vi "Pinholes.vi"(4 "Current Threshold [nA]":dbl, 5 "settling\ndelay":i32) -> (1 "excluded channels":i32[](array[numeric]), 2 "Current [nA]":dbl[](array[numeric]), 3 "Flag":i32[](array[numeric]))   [LabVIEW 2019]
uses:
  general_VIs/globals/QC_MeasurementSetup.vi
  InstrControl/Switching/Switching.lvclass
  InstrControl/SupplyControl/SupplyControl.lvclass
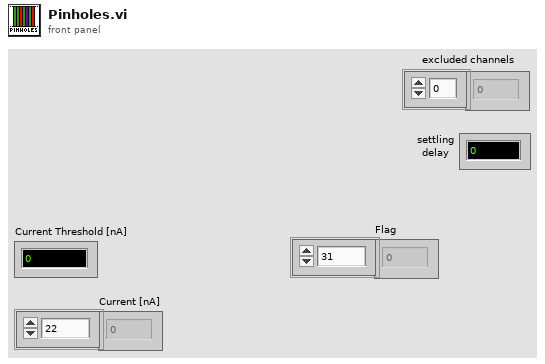
[diagram p1: front panel]
types:
  T1 = cluster{"Bias Supply":refnum<class "SupplyControl.lvclass">, "SMU":refnum<class "SupplyControl.lvclass">, "LCR":refnum<class "LCRControl.lvclass">, "Probe Card Channels":i32, "Bias Voltage [V]":dbl, "First strip":i32, "Last strip":i32, "Base Voltage [V]":dbl, "Base Ramp Step [V]":dbl, "Base Ramp Interval [ms]":u32, "High Voltage [V]":dbl, "High Ramp Step [V]":dbl, "High Ramp Interval [ms]":u32, "AC frequency [Hz]":i32, "AC amplitude [V]":dbl, "RC Configuration":u16, "Single Needle":bool, "Temperature Readout":enum16{"Read Arduino", "Enter manually"}, "Arduino":refnum<class "ArduinoControl.lvclass">, "Fraction of good strips [%]":dbl, "ProbeStation":refnum<class "ProbeStationControl.lvclass">, "Switching":refnum<class "Switching.lvclass">, "Matrix used?":bool, "Matrix X Channels":cluster{"Bias Supply / SMU LO":i32, "Bias Supply / SMU HI":i32, "CV Box LO":i32, "CV Box HI":i32, "CV Box LO IN":i32, "CV Box HI IN":i32, "Volt meter LO":i32, "Volt meter HI":i32, "Mux1 C1":i32, "Mux1 C2":i32, "Mux2 C1":i32, "Mux2 C2":i32}, "Pinholes Y/N":bool, "Capacitance Y/N":bool, "Resistance Y/N":bool, "Bias Supply Name":string, "SMU Name":string, "LCR Name":string}
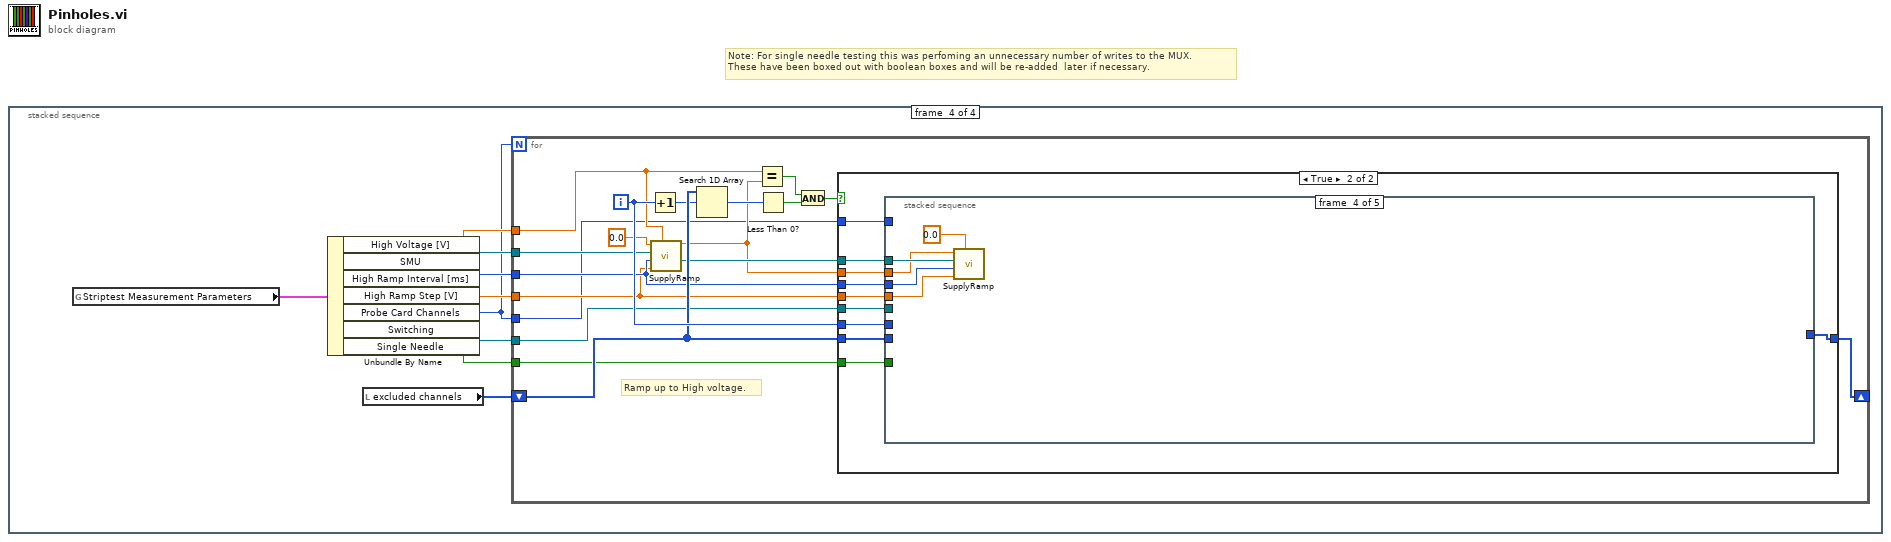
[diagram p0: block diagram]
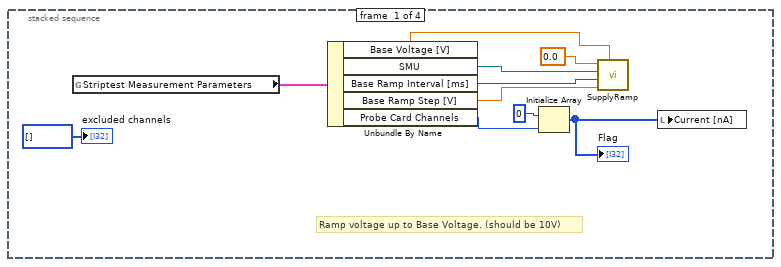
[diagram p2: hidden frame]
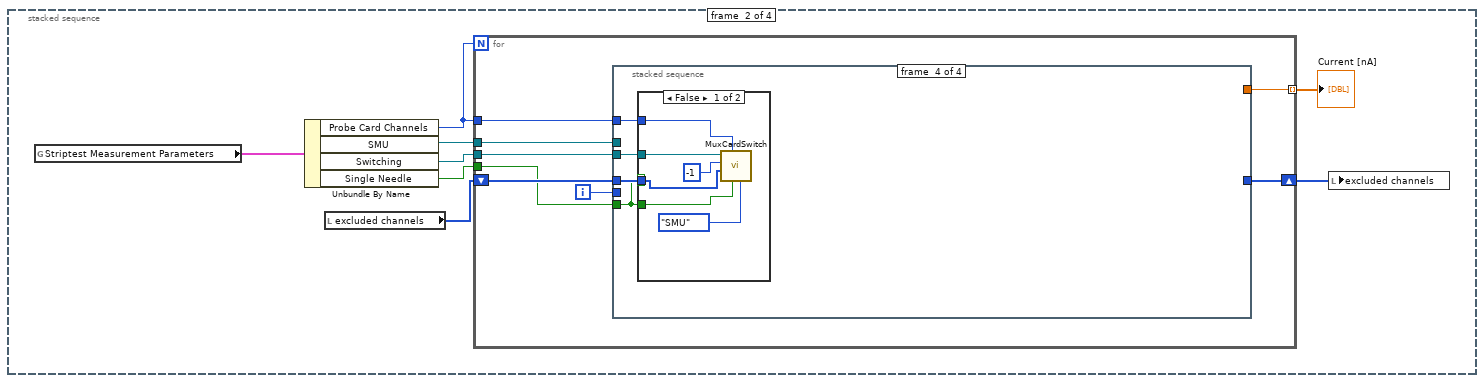
[diagram p3: hidden frame]
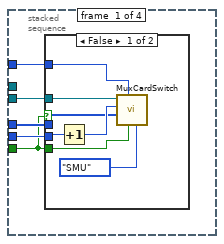
[diagram p4: hidden frame]
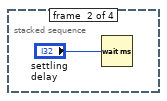
[diagram p6: hidden frame]
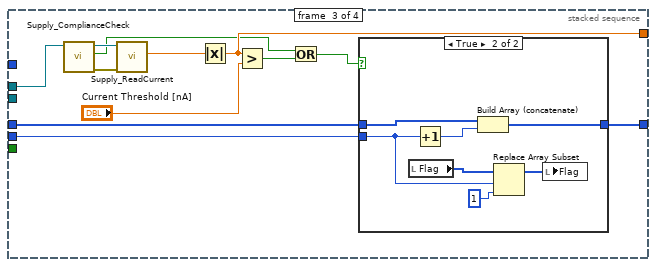
[diagram p7: hidden frame]
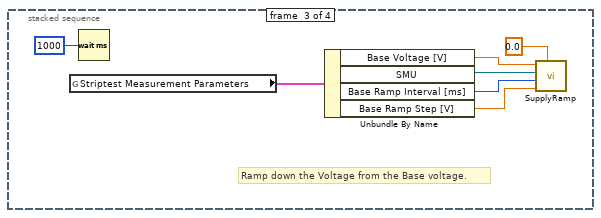
[diagram p10: hidden frame]
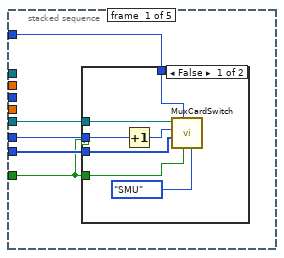
[diagram p12: hidden frame]
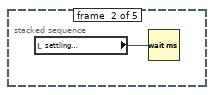
[diagram p14: hidden frame]
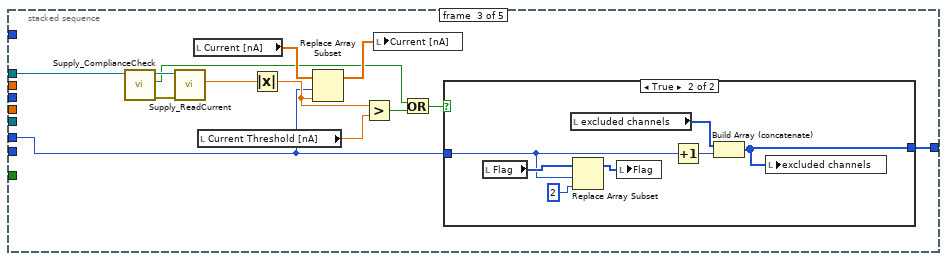
[diagram p15: hidden frame]
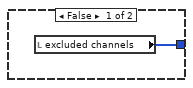
[diagram p16: hidden frame]
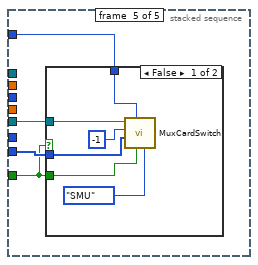
[diagram p17: hidden frame]
diagram:
  # "Note: For single needle testing this was perfoming an unnecessary number of writes to the MUX.\nThese have been boxed out with boolean boxes and will be re-added  later if necessary."
  n1 = stacked-sequence {
    frame #0 {
      # "Ramp voltage up to Base Voltage. (should be 10V)"
      n2 = global read "QC_MeasurementSetup.vi" "Striptest Measurement Parameters"() -> (w6:T1)
      n3 = Unbundle By Name(w6) -> ("Base Voltage [V]"=w5:dbl, "SMU"=w1:refnum<class "SupplyControl.lvclass">, "Base Ramp Interval [ms]"=w4:u32, "Base Ramp Step [V]"=w3:dbl, "Probe Card Channels"=w2:i32)
      n4 = Initialize Array(0, w2) -> (w7:i32[])
      "Flag" <- w7
      n5 = call "SupplyRamp.vi"("Requested Voltage"=w5, "Step Size"=w3, "Step Delay"=w4, "Supply IN"=w1, "Starting Voltage"=0.0) -> ()  [unwired: 3 in, 4 out]
      n6 = local write "Current [nA]"(w7) -> ()
      "excluded channels" <- i32[] []
    }
    frame #1 {
      n7 = global read "QC_MeasurementSetup.vi" "Striptest Measurement Parameters"() -> (w16:T1)
      n8 = Unbundle By Name(w16) -> ("Probe Card Channels"=w11:i32, "SMU"=w15:refnum<class "SupplyControl.lvclass">, "Switching"=w13:refnum<class "Switching.lvclass">, "Single Needle"=w12:bool)
      n9 = local read "excluded channels"() -> (w17:i32[])
      n10 = for {
        N: w11 -> [_]
        tunnel: w11 -> [w26]
        tunnel: [w25] -> w18 mode=indexing
        shift-right: [w22] -> w14
        shift-left: w17 -> [w24]
        tunnel: w13 -> [w19]
        tunnel: w12 -> [w21]
        tunnel: w15 -> [w20]
        i -> [w23]
        n11 = stacked-sequence {
          tunnel: w23 -> [w29 _ w40 _]
          tunnel: w26 -> [w31 _ _ w62]
          tunnel: w24 -> [w30 _ w42 w61]
          tunnel: [_ _ w47 _] -> w25
          tunnel: [_ _ w48 _] -> w22
          tunnel: w19 -> [w28 _ _ w63]
          tunnel: w21 -> [w27 _ _ w60]
          tunnel: w20 -> [_ _ w41 _]
          frame #0 {
            n12 = case shown="False" w27 {
              tunnel: w31 -> [w37 _]
              tunnel: w30 -> [w36 _]
              tunnel: w29 -> [w35 _]
              tunnel: w28 -> [w34 _]
              tunnel: w27 -> [w33 _]
              frame False {
                n13 = Increment(x=w35) -> (x+1=w38:i32)
                n14 = call-dynamic "MuxCardSwitch.vi"("Instrument"=enum16{"SMU", "LCR"}."SMU", "Single Needle"=w33, "Probe Card Channels"=w37, "disabled channels"=w36, "Switch to channel"=w38, "Switching in"=w34) -> ()  [unwired: 3 in, 3 out]
              }
              frame True {
              }
            }
          }
          frame #1 {
            n15 = Wait (ms)(milliseconds to wait="settling\ndelay") -> ()  [unwired: 1 out]
          }
          frame #2 {
            n16 = call-dynamic "Supply_ComplianceCheck.vi"("SupplyControl in"=w41) -> ("error out"=w46:errorcluster, "Compliance exceeded?"=w43:bool, "SupplyControl out"=w45:refnum<class "SupplyControl.lvclass">)  [unwired: 7 in, 1 out]
            n17 = call-dynamic "Supply_ReadCurrent.vi"("error in (no error)"=w46, "SupplyControl in"=w45) -> ("Current in nA"=w44:dbl)  [unwired: 7 in, 2 out]
            n18 = Absolute Value(x=w44) -> (abs(x)=w47:dbl)
            n19 = Greater?(x=w47, y="Current Threshold [nA]") -> (0:w49:bool)
            n20 = Or(x=w43, y=w49) -> (x .or. y?=w50:bool)
            n21 = case shown="True" w50 {
              tunnel: w42 -> [w52 w53]
              tunnel: [w52 w55] -> w48
              tunnel: w40 -> [_ w54]
              frame False {
              }
              frame True {
                n22 = local read "Flag"() -> (w59:i32[])
                n23 = Increment(x=w54) -> (x+1=w56:i32)
                n24 = Build Array (concatenate)(w53, w56) -> (w55:i32[])
                n25 = Replace Array Subset(array=w59, new element=1, index=w54) -> (w57:i32[])
                n26 = local write "Flag"(w57) -> ()
              }
            }
          }
          frame #3 {
            n27 = case shown="False" w60 {
              tunnel: w63 -> [w68 _]
              tunnel: w60 -> [w67 _]
              tunnel: w62 -> [w66 _]
              tunnel: w61 -> [w65 _]
              frame False {
                n28 = call-dynamic "MuxCardSwitch.vi"("Instrument"=enum16{"SMU", "LCR"}."SMU", "Single Needle"=w67, "Probe Card Channels"=w66, "disabled channels"=w65, "Switch to channel"=-1, "Switching in"=w68) -> ()  [unwired: 3 in, 3 out]
              }
              frame True {
              }
            }
          }
        }
      }
      "Current [nA]" <- w18
      n29 = local write "excluded channels"(w14) -> ()
    }
    frame #2 {
      # "Ramp down the Voltage from the Base voltage."
      n30 = global read "QC_MeasurementSetup.vi" "Striptest Measurement Parameters"() -> (w74:T1)
      n31 = Wait (ms)(milliseconds to wait=1000) -> ()  [unwired: 1 out]
      n32 = Unbundle By Name(w74) -> ("Base Voltage [V]"=w72:dbl, "SMU"=w73:refnum<class "SupplyControl.lvclass">, "Base Ramp Interval [ms]"=w71:u32, "Base Ramp Step [V]"=w70:dbl)
      n33 = call "SupplyRamp.vi"("Requested Voltage"=0.0, "Step Size"=w70, "Step Delay"=w71, "Supply IN"=w73, "Starting Voltage"=w72) -> ()  [unwired: 3 in, 4 out]
    }
    frame #3 {
      n34 = global read "QC_MeasurementSetup.vi" "Striptest Measurement Parameters"() -> (w84:T1)
      n35 = Unbundle By Name(w84) -> ("High Voltage [V]"=w83:dbl, "SMU"=w82:refnum<class "SupplyControl.lvclass">, "High Ramp Interval [ms]"=w81:u32, "High Ramp Step [V]"=w80:dbl, "Probe Card Channels"=w78:i32, "Switching"=w79:refnum<class "Switching.lvclass">, "Single Needle"=w77:bool)
      n36 = local read "excluded channels"() -> (w85:i32[])
      n37 = for {
        N: w78 -> [_]
        shift-right: [w103] -> _
        shift-left: w85 -> [w101]
        tunnel: w83 -> [w92]
        tunnel: w82 -> [w91]
        tunnel: w81 -> [w90]
        tunnel: w80 -> [w89]
        tunnel: w79 -> [w88]
        tunnel: w78 -> [w87]
        tunnel: w77 -> [w86]
        i -> [w102]
        # "Ramp up to High voltage."
        n38 = Increment(x=w102) -> (x+1=w100:i32)
        n39 = call "SupplyRamp.vi"("Requested Voltage"=w92, "Step Size"=w89, "Step Delay"=w90, "Supply IN"=w91, "Starting Voltage"=0.0) -> ("Supply OUT"=w94:refnum<class "SupplyControl.lvclass">, "Current Voltage"=w93:dbl)  [unwired: 3 in, 2 out]
        n40 = Search 1D Array(1D array=w101, element=w100) -> (index of element=w99:i32)  [unwired: 1 in]
        n41 = Equal?(x=w92, y=w93) -> (x = y?=w95:bool)
        n42 = Less Than 0?(x=w99) -> (x < 0?=w97:bool)
        n43 = And(x=w95, y=w97) -> (x .and. y?=w96:bool)
        n44 = case shown="True" w96 {
          tunnel: w101 -> [w104 w114]
          tunnel: w102 -> [_ w113]
          tunnel: [w104 w112] -> w103
          tunnel: w89 -> [_ w111]
          tunnel: w87 -> [_ w110]
          tunnel: w88 -> [_ w109]
          tunnel: w86 -> [_ w108]
          tunnel: w94 -> [_ w107]
          tunnel: w93 -> [_ w106]
          tunnel: w90 -> [_ w105]
          frame False {
          }
          frame True {
            n45 = stacked-sequence {
              tunnel: w113 -> [w118 _ w128 _ _]
              tunnel: w114 -> [w119 _ _ _ w155]
              tunnel: [_ _ w138 _ _] -> w112
              tunnel: w111 -> [_ _ _ w149 _]
              tunnel: w110 -> [w117 _ _ _ w156]
              tunnel: w109 -> [w116 _ _ _ w157]
              tunnel: w108 -> [w115 _ _ _ w154]
              tunnel: w107 -> [_ _ w130 w152 _]
              tunnel: w106 -> [_ _ _ w151 _]
              tunnel: w105 -> [_ _ _ w150 _]
              frame #0 {
                n46 = case shown="False" w115 {
                  tunnel: w119 -> [w125 _]
                  tunnel: w118 -> [w124 _]
                  tunnel: w117 -> [w123 _]
                  tunnel: w116 -> [w122 _]
                  tunnel: w115 -> [w121 _]
                  frame False {
                    n47 = Increment(x=w124) -> (x+1=w126:i32)
                    n48 = call-dynamic "MuxCardSwitch.vi"("Instrument"=enum16{"SMU", "LCR"}."SMU", "Single Needle"=w121, "Probe Card Channels"=w123, "disabled channels"=w125, "Switch to channel"=w126, "Switching in"=w122) -> ()  [unwired: 3 in, 3 out]
                  }
                  frame True {
                  }
                }
              }
              frame #1 {
                n49 = local read "settling\ndelay"() -> (w127:i32)
                n50 = Wait (ms)(milliseconds to wait=w127) -> ()  [unwired: 1 out]
              }
              frame #2 {
                n51 = call-dynamic "Supply_ComplianceCheck.vi"("SupplyControl in"=w130) -> ("error out"=w132:errorcluster, "Compliance exceeded?"=w129:bool, "SupplyControl out"=w133:refnum<class "SupplyControl.lvclass">)  [unwired: 7 in, 1 out]
                n52 = call-dynamic "Supply_ReadCurrent.vi"("error in (no error)"=w132, "SupplyControl in"=w133) -> ("Current in nA"=w131:dbl)  [unwired: 7 in, 2 out]
                n53 = local read "Current [nA]"() -> (w135:dbl[])
                n54 = local read "Current Threshold [nA]"() -> (w137:dbl)
                n55 = Absolute Value(x=w131) -> (abs(x)=w134:dbl)
                n56 = Replace Array Subset(array=w135, new element=w134, index=w128) -> (w136:dbl[])
                n57 = Greater?(x=w134, y=w137) -> (0:w139:bool)
                n58 = local write "Current [nA]"(w136) -> ()
                n59 = Or(x=w129, y=w139) -> (x .or. y?=w140:bool)
                n60 = case shown="True" w140 {
                  tunnel: w128 -> [_ w144]
                  tunnel: [w141 w142] -> w138
                  frame False {
                    n61 = local read "excluded channels"() -> (w141:i32[])
                  }
                  frame True {
                    n62 = local read "Flag"() -> (w148:i32[])
                    n63 = local read "excluded channels"() -> (w145:i32[])
                    n64 = Replace Array Subset(array=w148, new element=2, index=w144) -> (w146:i32[])
                    n65 = local write "Flag"(w146) -> ()
                    n66 = Increment(x=w144) -> (x+1=w143:i32)
                    n67 = Build Array (concatenate)(w145, w143) -> (w142:i32[])
                    n68 = local write "excluded channels"(w142) -> ()
                  }
                }
              }
              frame #3 {
                n69 = call "SupplyRamp.vi"("Requested Voltage"=0.0, "Step Size"=w149, "Step Delay"=w150, "Supply IN"=w152, "Starting Voltage"=w151) -> ()  [unwired: 3 in, 4 out]
              }
              frame #4 {
                n70 = case shown="False" w154 {
                  tunnel: w157 -> [w162 _]
                  tunnel: w154 -> [w161 _]
                  tunnel: w156 -> [w160 _]
                  tunnel: w155 -> [w159 _]
                  frame False {
                    n71 = call-dynamic "MuxCardSwitch.vi"("Instrument"=enum16{"SMU", "LCR"}."SMU", "Single Needle"=w161, "Probe Card Channels"=w160, "disabled channels"=w159, "Switch to channel"=-1, "Switching in"=w162) -> ()  [unwired: 3 in, 3 out]
                  }
                  frame True {
                  }
                }
              }
            }
          }
        }
      }
    }
  }
